vi "Load config.vi"(8 "error in (no error)":errorcluster) -> (0 "error out":errorcluster, 3 "Config":T1={"Arduino port"="COM4", "Starting angle M1"=0.0, "Starting angle M2"=0.0})   [LabVIEW 2025]
uses:
  Config -- cluster.ctl
  <vilib>/Utility/config.llb/Read Key (String).vi
  <vilib>/Utility/config.llb/Read Key (Double).vi
  <vilib>/Utility/config.llb/NI_LVConfig.lvlib
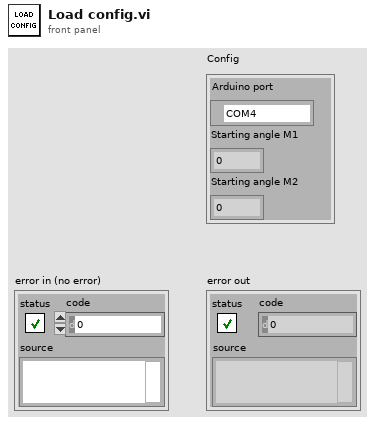
[diagram p1: front panel]
types:
  T1 = typedef "Config -- cluster.ctl" = cluster{"Arduino port":refnum<visa-resource-name>, "Starting angle M1":dbl, "Starting angle M2":dbl}
  T2 = typedef "NI_LVConfig.lvlib/Config Data RefNum.ctl" = refnum<k1>
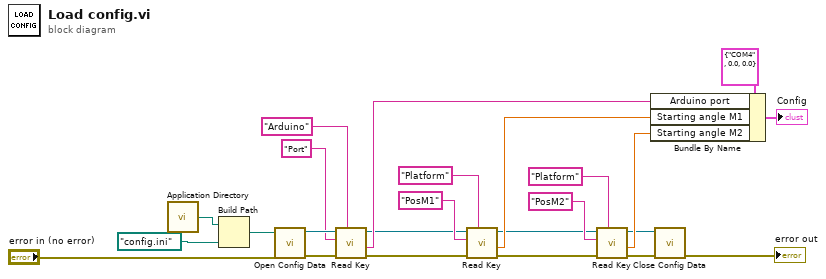
[diagram p0: block diagram]
diagram:
  n1 = call <vilib>:"Application Directory.vi"() -> ("Application Directory"=w17:path)
  n2 = Build Path(base path=w17, name or relative path=path "config.ini") -> (appended path=w15:path)
  n3 = call <vilib>:"Open Config Data.vi"("error in (no error)"="error in (no error)", "configuration file path"=w15) -> ("error out"=w14:errorcluster, "refnum"=w13:T2)  [unwired: 7 in, 1 out]
  n4 = call-poly <vilib>:"Read Key.vi"("section"="Arduino", "error in (no error)"=w14, "key"="Port", "refnum"=w13) -> ("error out"=w10:errorcluster, "value"=w22:string, "refnum out"=w7:T2)  [unwired: 4 in, 1 out]
  n5 = call-poly <vilib>:"Read Key.vi"("section"="Platform", "error in (no error)"=w10, "key"="PosM1", "refnum"=w7) -> ("error out"=w3:errorcluster, "value"=w23:dbl, "refnum out"=w4:T2)  [unwired: 4 in, 1 out]
  n6 = call-poly <vilib>:"Read Key.vi"("section"="Platform", "error in (no error)"=w3, "key"="PosM2", "refnum"=w4) -> ("error out"=w2:errorcluster, "value"=w24:dbl, "refnum out"=w1:T2)  [unwired: 4 in, 1 out]
  n7 = Bundle By Name(cluster=T1 {"Arduino port"="COM4", "Starting angle M1"=0.0, "Starting angle M2"=0.0} ("Config"), "Arduino port"=w22, "Starting angle M1"=w23, "Starting angle M2"=w24) -> (→"Config":T1)
  n8 = call <vilib>:"Close Config Data.vi"("error in (no error)"=w2, "refnum"=w1) -> ("error out"=→"error out":errorcluster)  [unwired: 8 in, 1 out]
